vi "Saving_Data.vi"(2 "error in":errorcluster, 3 "report in":refnum<class "NI_report.lvclass">, 5 "Current":dbl, 6 "Input":string[][](array[string]), 7 "Watt":dbl, 8 "Voltage":dbl, 9 "RPM":dbl, 10 "Iteration":i32, 11 "Path":path) -> (0 "error out":errorcluster, 1 "report out":refnum<class "NI_report.lvclass">, 4 "output":string[][](array[string]))   [LabVIEW 2013, in "Test_Libraries.lvlib"]
uses:
  Proyecto/Test_Libraries.lvlib
  <vilib>/Utility/NIReport.llb/Excel/NI_Excel.lvclass
  <vilib>/Utility/NIReport.llb/NI_report.lvclass
  <vilib>/Utility/NIReport.llb/Append Text Table to Report (wrap).vi
  <vilib>/addons/_office/_exclsub.llb/font.ctl
  <vilib>/addons/_office/NI_ReportGenerationToolkit.lvlib
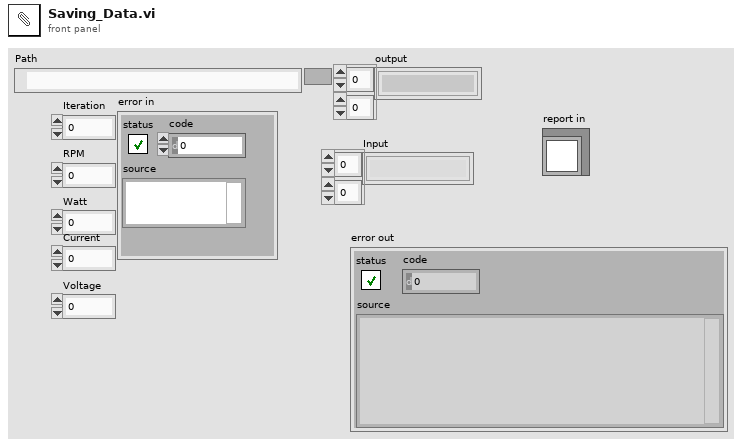
[diagram p1: front panel]
types:
  T1 = typedef "NI_ReportGenerationToolkit.lvlib/font.ctl" = cluster{"font name":string, "font size":dbl, "bold":u16, "italic":u16, "underline":u16, "strike through":u16, "font color":u32}
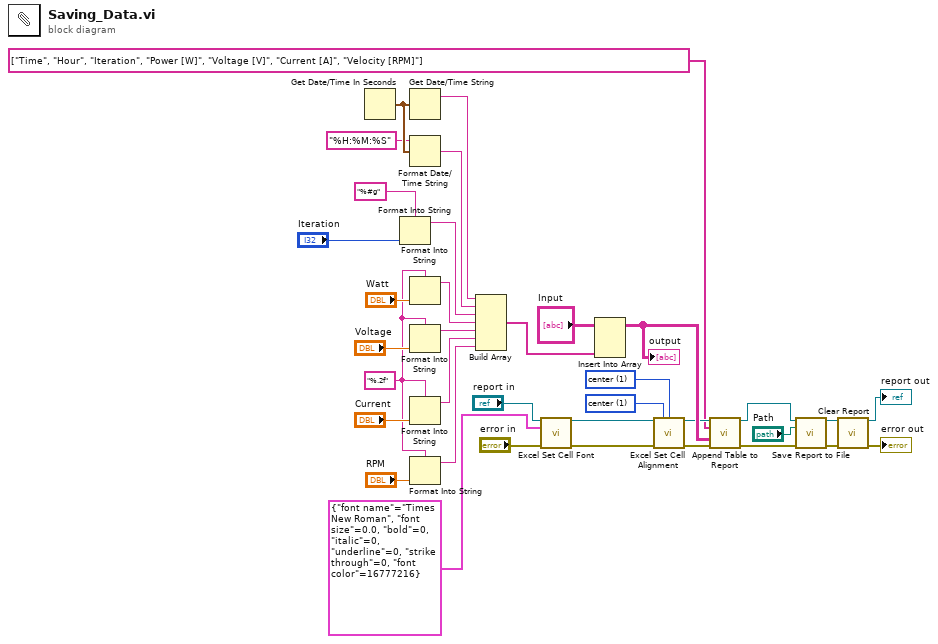
[diagram p0: block diagram]
diagram:
  w20 = "%.2f" ("format string")
  w17 = 1 items=["left", "center", "right"] ("horizontal alignment (left)")
  w18 = 1 items=["top", "center", "bottom"] ("vertical alignment (top)")
  n1 = Get Date/Time In Seconds() -> (seconds since 1Jan1904=w33:timestamp)
  n2 = Format Into String(format string="%#g", "Iteration") -> (resulting string=w28:string)  [unwired: 2 in, 1 out]
  n3 = Get Date/Time String(seconds (now)=w33) -> (date string=w34:string)  [unwired: 2 in, 1 out]
  n4 = Format Date/Time String(time format string (%c)="%H:%M:%S", seconds (now)=w33) -> (date/time string=w35:string)  [unwired: 1 in]
  n5 = Format Into String(format string=w20, "Watt") -> (resulting string=w29:string)  [unwired: 2 in, 1 out]
  n6 = Format Into String(format string=w20, "Voltage") -> (resulting string=w30:string)  [unwired: 2 in, 1 out]
  n7 = Format Into String(format string=w20, "Current") -> (resulting string=w31:string)  [unwired: 2 in, 1 out]
  n8 = Format Into String(format string=w20, "RPM") -> (resulting string=w32:string)  [unwired: 2 in, 1 out]
  n9 = Build Array(w34, w35, w28, w29, w30, w31, w32) -> (w36:string[])
  n10 = call <vilib>:"Excel Set Cell Font.vi"("report in"="report in", "font"=T1 {"font name"="Times New Roman", "font size"=0.0, "bold"=0, "italic"=0, "underline"=0, "strike through"=0, "font color"=16777216}, "error in (no error)"="error in") -> ("report out"=w5:refnum<class "NI_report.lvclass">, "error out"=w6:errorcluster)  [unwired: 11 in]
  n11 = Insert Into Array(array="Input", new element=w36) -> (w13:string[][])  [unwired: 2 in]
  "output" <- w13
  n12 = call <vilib>:"Excel Set Cell Alignment.vi"("report in"=w5, "vertical alignment (top)"=w18, "horizontal alignment (left)"=w17, "error in (no error)"=w6) -> ("report out"=w10:refnum<class "NI_report.lvclass">, "error out"=w9:errorcluster)  [unwired: 10 in]
  n13 = call-poly <vilib>:"Append Table to Report.vi"("report in"=w10, "column headers"=string[] ["Time", "Hour", "Iteration", "Power [W]", "Voltage [V]", "Current [A]", "Velocity [RPM]"] ("row headers"), "text data"=w13, "error in (no error)"=w9) -> ("report out"=w8:refnum<class "NI_report.lvclass">, "error out"=w7:errorcluster)  [unwired: 8 in, 2 out]
  n14 = call-dynamic "Save Report to File.vi"("report in"=w8, "report file path"="Path", "error in (no error)"=w7) -> ("report out"=w16:refnum<class "NI_report.lvclass">, "error out"=w15:errorcluster)  [unwired: 11 in]
  n15 = call-dynamic "Clear Report.vi"("report in"=w16, "error in (no error)"=w15) -> ("report out"=→"report out":refnum<class "NI_report.lvclass">, "error out"=→"error out":errorcluster)  [unwired: 12 in]
